vi "Enqueue_Acquisition.vi"() -> ()   [LabVIEW 2022 SP3]
uses:
  <vilib>/userdefined/High Color/IMAQdx.ctl
  <vilib>/vision/driver/IMAQdx.llb/IMAQdx Acquisition Mode.ctl
  <vilib>/vision/driver/NI_Vision_Acquisition_Software.lvlib
panel:
  out "Image":T1(plugin-control)
  out "Buffer Number Out":u32
  in  "stop":bool
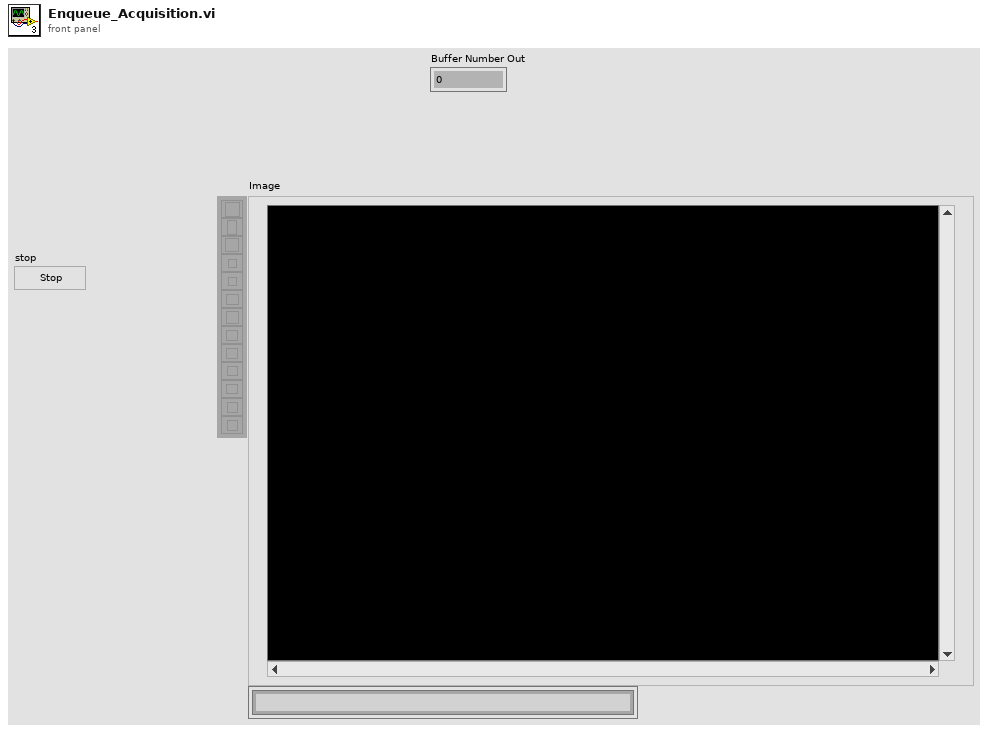
[diagram p1: front panel]
types:
  T1 = typedef "IMAQ Image.ctl" = refnum<image>
  T2 = typedef "Image Type" = u32
  T3 = typedef "NI_Vision_Acquisition_Software.lvlib/IMAQdx Acquisition Mode.ctl" = enum32{"One Shot", "Continuous"}
  T4 = typedef "IMAQdx.ctl" = refnum<k21>
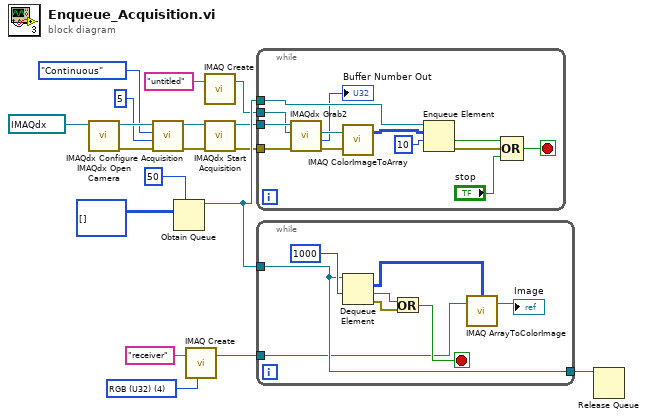
[diagram p0: block diagram]
diagram:
  w1 = T2 4 items=["Grayscale (U8)", "Grayscale (I16)", "Grayscale (SGL)", "Complex (CSG)", "RGB (U32)", "HSL (U32)", "RGB (U64)", "Grayscale (U16)"] ("Image Type")
  n1 = call <vilib>:"IMAQdx Open Camera.vi"("Session In"=T4 "cam3") -> ("error out"=w12:errorcluster, "Session Out"=w13:T4)  [unwired: 9 in]
  n2 = call <vilib>:"IMAQdx Configure Acquisition.vi"("error in"=w12, "Number of Buffers"=u32 5, "Continuous?"=IMAQdx_Acquisition_Mode."Continuous", "Session In"=w13) -> ("error out"=w5:errorcluster, "Session Out"=w16:T4)  [unwired: 6 in]
  n3 = Obtain Queue(max queue size (-1, unlimited)=50, element data type=u32[][] [] ("Image Pixels (U32)")) -> (queue out=w17:refnum<queue>)  [unwired: 3 in, 2 out]
  n4 = call "IMAQ Create"("Image Name"="receiver", "Image Type"=w1) -> ("New Image"=w2:T1)  [unwired: 3 in, 1 out]
  n5 = call "IMAQ Create"("Image Name"="untitled") -> ("New Image"=w14:T1)  [unwired: 4 in, 1 out]
  n6 = call <vilib>:"IMAQdx Start Acquisition.vi"("error in"=w5, "Session In"=w16) -> ("error out"=w4:errorcluster, "Session Out"=w6:T4)  [unwired: 8 in]
  n7 = while {
    tunnel: w17 -> [w31]
    tunnel: w6 -> [w28]
    tunnel: w14 -> [w27]
    tunnel: w4 -> [w26]
    stop <- w23 stop-if-true
    n8 = call <vilib>:"IMAQdx Grab2.vi"("error in"=w26, "Image In"=w27, "Session In"=w28) -> ("error out"=w29:errorcluster, "Buffer Number Out"=→"Buffer Number Out":u32, "Image Out"=w30:T1)  [unwired: 5 in, 1 out]
    n9 = call "IMAQ ColorImageToArray"("Image"=w30, "error in (no error)"=w29) -> ("Image Pixels (U32)"=w19:u32[][])  [unwired: 2 in, 2 out]
    n10 = Enqueue Element(queue=w31, element=w19, timeout in ms (-1)=10) -> (timed out?=w25:bool, error out=w24:errorcluster)  [unwired: 1 in, 1 out]
    n11 = Compound Arithmetic op=OR(w25, w24, "stop") -> (w23:bool)
  }
  n12 = while {
    tunnel: w17 -> [w37]
    tunnel: [w37] -> w7
    tunnel: w2 -> [w33]
    stop <- w36 stop-if-true
    n13 = Dequeue Element(queue=w37, timeout in ms (-1)=1000) -> (element=w34:u32[][], timed out?=w38:bool, error out=w35:errorcluster)  [unwired: 1 in, 1 out]
    n14 = Or(x=w38, y=w35) -> (x .or. y?=w36:bool)
    n15 = call "IMAQ ArrayToColorImage"("Image Pixels (U32)"=w34, "Image"=w33) -> ("Image Out"=→"Image":T1)  [unwired: 3 in, 1 out]
  }
  n16 = Release Queue(queue=w7) -> ()  [unwired: 2 in, 3 out]
